vi "2D数组水平镜像[TimeStamp].vi"(8 "error in (no error)":errorcluster caption="错误输入（无错误）", 11 "数组":timestamp[][](array[timestamp])) -> (0 "error out":errorcluster caption="错误输出", 3 "水平镜像":timestamp[][](array[timestamp]))   [LabVIEW 2012]
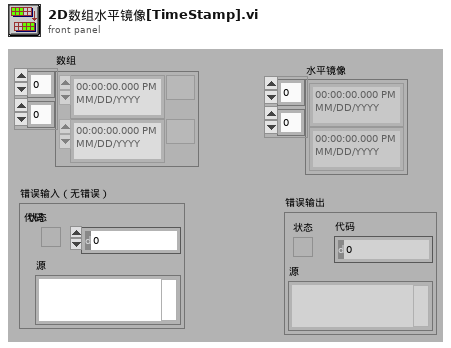
[diagram p1: front panel]
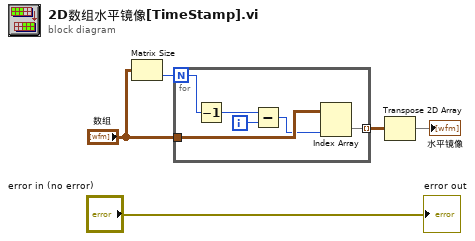
[diagram p0: block diagram]
diagram:
  n1 = Matrix Size(0:"数组") -> (2:w2:i32)  [unwired: 1 out]
  n2 = for {
    N: w2 -> [w11]
    tunnel: "数组" -> [w8]
    tunnel: [w7] -> w3 mode=indexing
    i -> [w9]
    n3 = Decrement(x=w11) -> (x-1=w10:i32)
    n4 = Subtract(x=w10, y=w9) -> (x-y=w6:i32)
    n5 = Index Array(array=w8, index (col)=w6) -> (element=w7:timestamp[])  [unwired: 1 in]
  }
  n6 = Transpose 2D Array(2D array=w3) -> (transposed array=→"水平镜像":timestamp[][])
  "error out" <- "error in (no error)"
